vi "Channel Validation.vi"(11 "User Defined Channels":i32[](array[numeric])) -> (2 "Chl Valid?":bool)   [LabVIEW 2021]
doc: "This VI helps to check if user defined channels are valid."
panel:
  out "Chl Duplicate":bool
  out "Chl Out of Range":bool
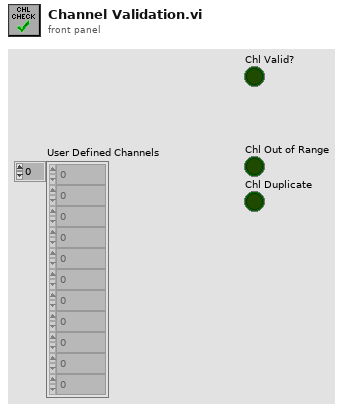
[diagram p1: front panel]
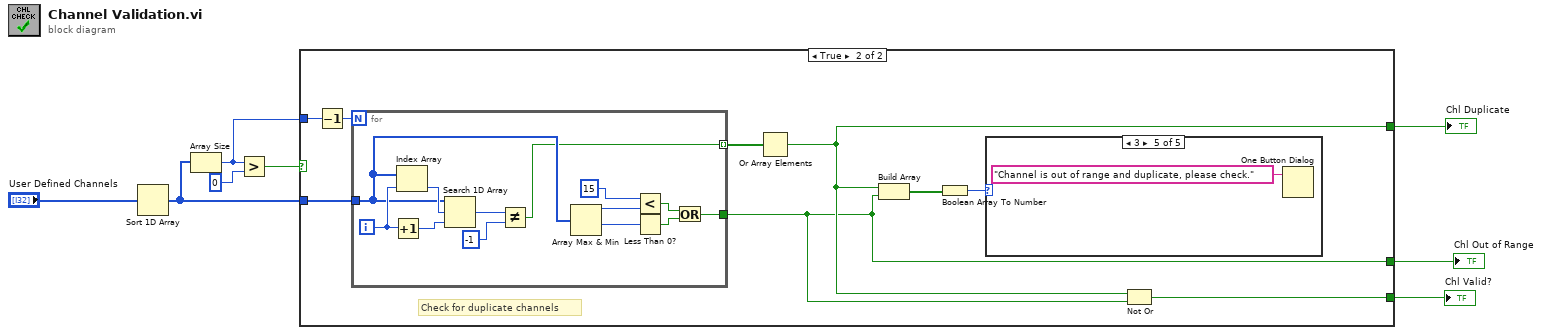
[diagram p0: block diagram]
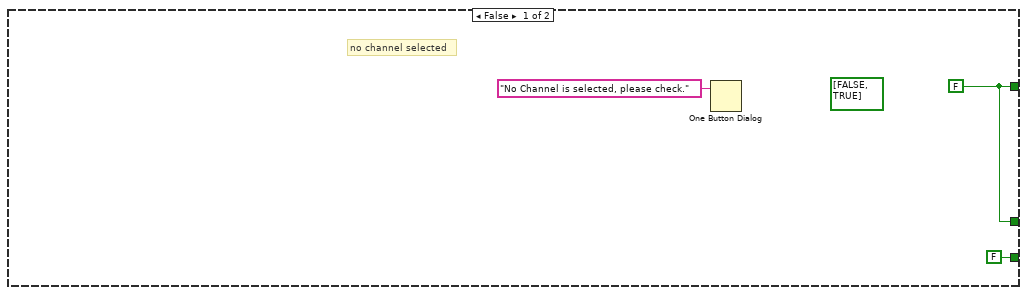
[diagram p2: hidden frame]
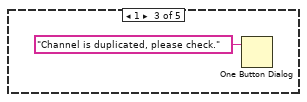
[diagram p5: hidden frame]
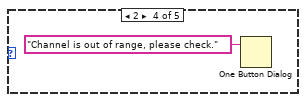
[diagram p6: hidden frame]
diagram:
  n1 = Sort 1D Array(array="User Defined Channels") -> (sorted array=w5:i32[])
  n2 = Array Size(array=w5) -> (size(s)=w6:i32)
  n3 = Greater?(x=w6, y=0) -> (0:w7:bool)
  n4 = case shown="True" w7 {
    tunnel: w6 -> [_ w20]
    tunnel: w5 -> [_ w18]
    tunnel: [w10 w14] -> w3
    tunnel: [w10 w13] -> w2
    tunnel: [FALSE w12] -> w1
    frame False {
      (unwired) bool[] [FALSE, TRUE]
      w10 = FALSE
      # "no channel selected"
      n5 = One Button Dialog(message="No Channel is selected, please check.") -> ()  [unwired: 1 in, 1 out]
    }
    frame True {
      # "Check for duplicate channels"
      n6 = Decrement(x=w20) -> (x-1=w19:i32)
      n7 = for {
        N: w19 -> [_]
        tunnel: w18 -> [w26]
        tunnel: [w25] -> w17 mode=indexing
        tunnel: [w24] -> w13
        i -> [w36]
        n8 = Increment(x=w36) -> (x+1=w35:i32)
        n9 = Index Array(array=w26, index=w36) -> (element=w34:i32)
        n10 = Search 1D Array(1D array=w26, element=w34, start index (0)=w35) -> (index of element=w33:i32)
        n11 = Not Equal?(x=w33, y=-1) -> (x != y?=w25:bool)
        n12 = Array Max & Min(array=w26) -> (max value=w28:i32, min value=w29:i32)  [unwired: 2 out]
        n13 = Less?(x=15 ("Max channel"), y=w28) -> (x < y?=w31:bool)
        n14 = Less Than 0?(x=w29) -> (x < 0?=w30:bool)
        n15 = Or(x=w31, y=w30) -> (x .or. y?=w24:bool)
      }
      n16 = Or Array Elements(Boolean array=w17) -> (logical OR=w14:bool)
      n17 = Build Array(w14, w13) -> (w15:bool[])
      n18 = Boolean Array To Number(Boolean array=w15) -> (number=w16:u32)
      n19 = case shown="3" w16 {
        frame Default {
        }
        frame 0 {
        }
        frame 1 {
          n20 = One Button Dialog(message="Channel is duplicated, please check.") -> ()  [unwired: 1 in, 1 out]
        }
        frame 2 {
          n21 = One Button Dialog(message="Channel is out of range, please check.") -> ()  [unwired: 1 in, 1 out]
        }
        frame 3 {
          n22 = One Button Dialog(message="Channel is out of range and duplicate, please check.") -> ()  [unwired: 1 in, 1 out]
        }
      }
      n23 = Not Or(1:w13, 2:w14) -> (0:w12:bool)
    }
  }
  "Chl Out of Range" <- w2
  "Chl Valid?" <- w1
  "Chl Duplicate" <- w3
